vi "StartStop Getting Joystick Update.vi"(8 "error in (no error)":errorcluster, 10 "Start?":bool, 11 "RPI.SenseHat.Actor in":refnum<class "RPI.SenseHat.Actor.lvclass">) -> (0 "error out":errorcluster, 3 "RPI.SenseHat.Actor out":refnum<class "RPI.SenseHat.Actor.lvclass">)   [LabVIEW 2020, in "RPI.SenseHat.Actor.lvlib" / "RPI.SenseHat.Actor.lvclass"]
uses:
  RPI.SenseHat.Actor.lvclass
  <vilib>/ActorFramework/Time-Delayed Send Message/Time-Delay Override Options.ctl
  RPI.SenseHat.Actor.lvclass/RPI.SenseHat.Actor.ctl
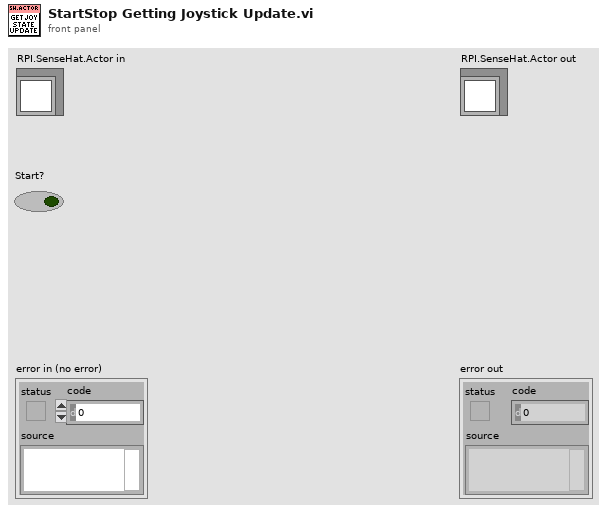
[diagram p1: front panel]
types:
  T1 = typedef "Time-Delay Override Options.ctl" = enum16{"Send next copy now", "Skip next scheduled copy", "Send next copy now and stop all further copies", "Stop all further copies"}
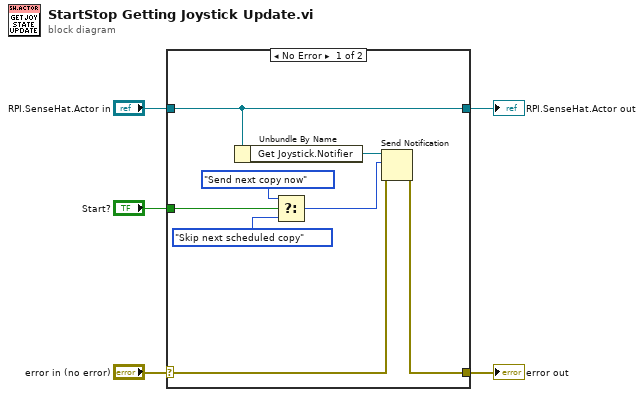
[diagram p0: block diagram]
diagram:
  n1 = case shown="No Error" "error in (no error)" {
    selector: "error in (no error)" -> [w11 w15]
    tunnel: [w10 w15] -> w4
    tunnel: [w13 w14] -> w2
    tunnel: "RPI.SenseHat.Actor in" -> [w13 w14]
    tunnel: "Start?" -> [w9 _]
    frame No Error {
      n2 = Unbundle By Name(w13) -> ("Get Joystick.Notifier"=w12:refnum<notifier>)
      n3 = Select(t=Time-Delay_Override_Options."Send next copy now" ("notification"), s=w9, f=Time-Delay_Override_Options."Skip next scheduled copy" ("notification")) -> (s? t:f=w6:T1)
      n4 = Send Notification(notification=w6, notifier=w12, error in (no error)=w11) -> (error out=w10:errorcluster)  [unwired: 1 out]
    }
    frame Error {
    }
  }
  "error out" <- w4
  "RPI.SenseHat.Actor out" <- w2
